vi "file -- list data files in mmddyy folder -- V2.vi"(11 "<mmddyy> folder path":path) -> (1 "Array":T1(array[cluster]))   [LabVIEW 2021]
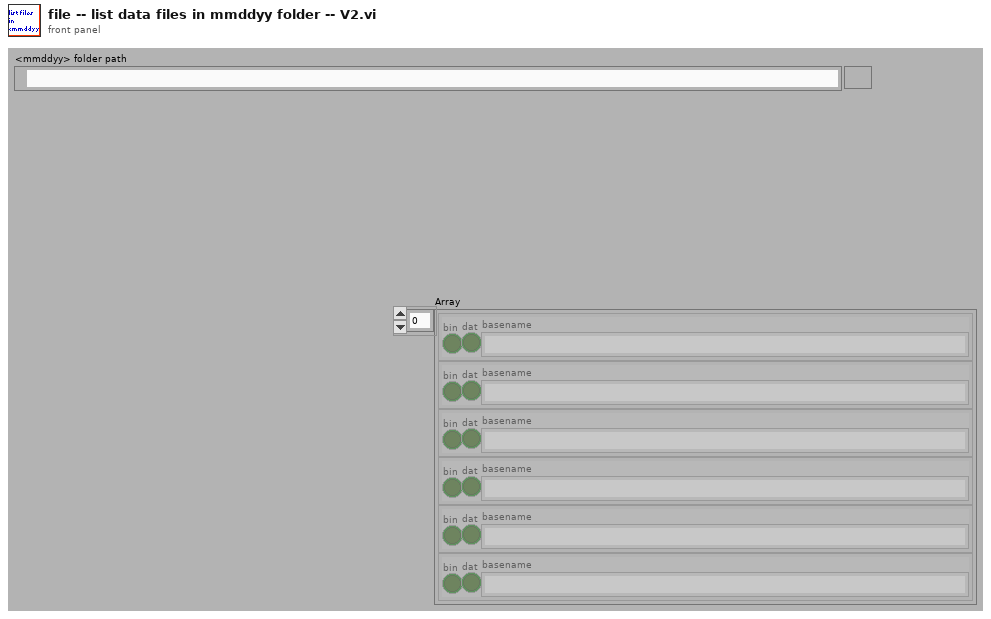
[diagram p1: front panel]
types:
  T1 = cluster{"basename":string, "dat":bool, "bin":bool}[]
  T2 = cluster{"basename":string, "dat":bool, "bin":bool}
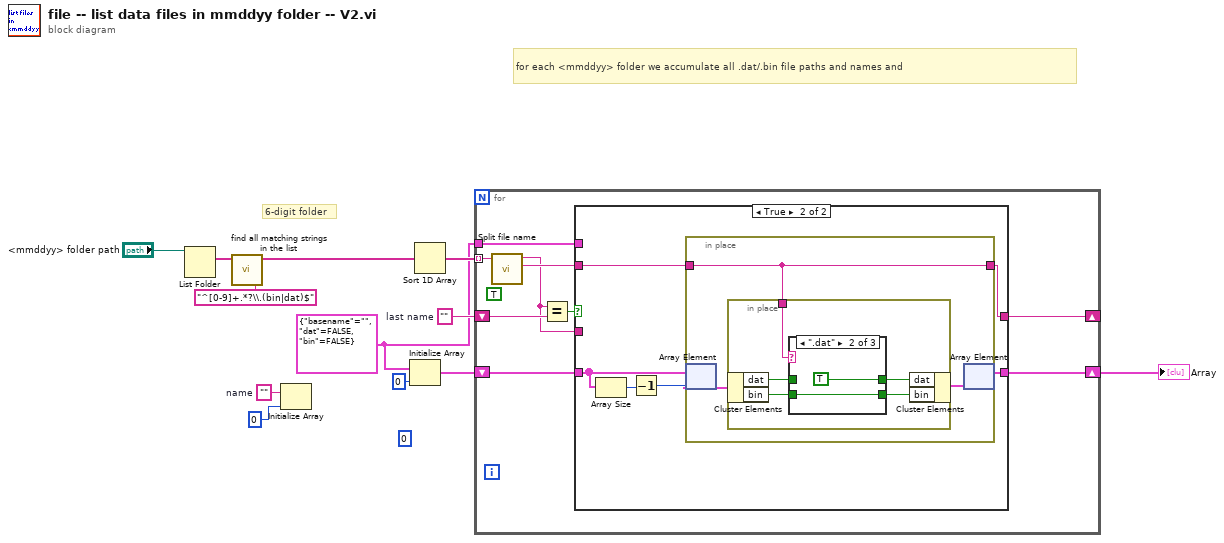
[diagram p0: block diagram]
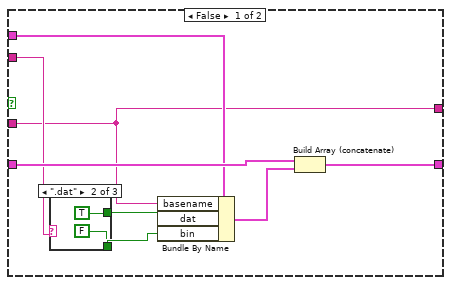
[diagram p2: hidden frame]
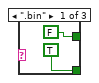
[diagram p3: hidden frame]
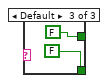
[diagram p4: hidden frame]
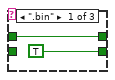
[diagram p5: hidden frame]
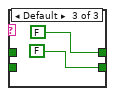
[diagram p6: hidden frame]
diagram:
  (unwired) 0
  w2 = ""  # last name
  w1 = T2 {"basename"="", "dat"=FALSE, "bin"=FALSE}
  w8 = ""  # name
  # "6-digit folder"
  # "for each <mmddyy> folder we accumulate all .dat/.bin file paths and names and"
  n1 = List Folder(path="<mmddyy> folder path") -> (filenames=w12:string[])  [unwired: 3 in, 3 out]
  n2 = call "find all matching strings in the list.vi"("regular expression"="^[0-9]+.*?\\.(bin|dat)$" ("pattern"), "strings"=w12) -> ("list of matching strings"=w6:string[])  [unwired: 7 in, 2 out]
  n3 = Initialize Array(w8, 0) -> ()  [unwired: 1 out]
  n4 = Initialize Array(w1, 0) -> (w4:T1)
  n5 = Sort 1D Array(array=w6) -> (sorted array=w5:string[])
  n6 = for {
    tunnel: w5 -> [w21] mode=indexing
    shift-right: [w13] -> w3
    shift-left: w4 -> [w18]
    shift-right: [w16] -> _
    shift-left: w2 -> [w20]
    tunnel: w1 -> [w15]
    (unwired) TRUE ("exact match")
    n7 = call "Split file name.vi"("file name"=w21) -> ("extension"=w17:string, "name"=w14:string)  [unwired: 8 in, 1 out]
    n8 = Equal?(x=w14, y=w20) -> (x = y?=w19:bool)
    n9 = case shown="True" w19 {
      tunnel: w18 -> [w28 w39]
      tunnel: w17 -> [w25 w38]
      tunnel: [w29 w36] -> w13
      tunnel: [w22 w37] -> w16
      tunnel: w15 -> [w24 _]
      tunnel: w14 -> [w22 _]
      frame False {
        n10 = case shown="\".dat\"" w25 {
          tunnel: [FALSE ("quote specials") TRUE ("quote specials") FALSE ("quote specials")] -> w27
          tunnel: [TRUE ("quote specials") FALSE ("quote specials") FALSE ("quote specials")] -> w26
          frame ".bin" {
          }
          frame ".dat" {
          }
          frame Default {
          }
        }
        n11 = Bundle By Name(cluster=w24, "basename"=w22, "dat"=w27, "bin"=w26) -> (w23:T2)
        n12 = Build Array (concatenate)(w28, w23) -> (w29:T1)
      }
      frame True {
        n13 = Array Size(array=w39) -> (size(s)=w41:i32)
        n14 = Decrement(x=w41) -> (x-1=w40:i32)
        n15 = in-place {
          in-place-border: w38 -> [w42]
          in-place-border: [w42] -> w37
          n16 = in-place-array #1(w39, w40) -> (w44:T2)
          n17 = in-place {
            in-place-border: w42 -> [w49]
            n18 = in-place-cluster #2(w44) -> ("dat"=w45:bool, "bin"=w46:bool)
            n19 = case shown="\".dat\"" w49 {
              tunnel: [w50 TRUE ("quote specials") FALSE ("quote specials")] -> w48
              tunnel: [TRUE ("quote specials") w52 FALSE ("quote specials")] -> w47
              tunnel: w46 -> [_ w52 _]
              tunnel: w45 -> [w50 _ _]
              frame ".bin" {
              }
              frame ".dat" {
              }
              frame Default {
              }
            }
            n20 = in-place-cluster #2("dat"=w48, "bin"=w47) -> (w43:T2)
          }
          n21 = in-place-array #1(w43) -> (w36:T1)  [unwired: 1 out]
        }
      }
    }
  }
  "Array" <- w3
